vi "Actor Core.vi"(8 "error in":errorcluster, 11 "Sequence Controller in":refnum<class "Sequence Controller.lvclass">) -> (0 "error out":errorcluster, 3 "Actor out":refnum<class "Actor.lvclass">)   [LabVIEW 2024, in "Sequence Controller.lvclass"]
doc: "(<B>Filename</B>: Actor Framework.lvlib:Actor.lvclass:Actor Core.vi)\n\nReceives messages to the actor, reacts to them, and initiates any error handling that may shut the actor down.\n\nDescendant classes may override this VI to append parallel tasks for the actor to complete while it handles messages. Overrides use the Call Parent Method node."
uses:
  Sequence Controller.lvclass
  Sequence Controller.lvclass/Sequence Controller.ctl
  <vilib>/ActorFramework/Actor/Actor.lvclass
  Sequence Elements/Sequence Element Messages/Items Mouse Click Msg/Items Mouse Click Msg.lvclass
  Template Module Messages/Open Item Msg/Open Item Msg.lvclass
  Sequence Controller Messages/Remove Sequence Element Msg/Remove Sequence Element Msg.lvclass
  Process Controller/Process Controller.lvclass
panel:
  in  "Remove Button":bool
  in  "Add Button":bool
  in  "Items":i32(listbox)
  in  "Measure sequence":string(tree)
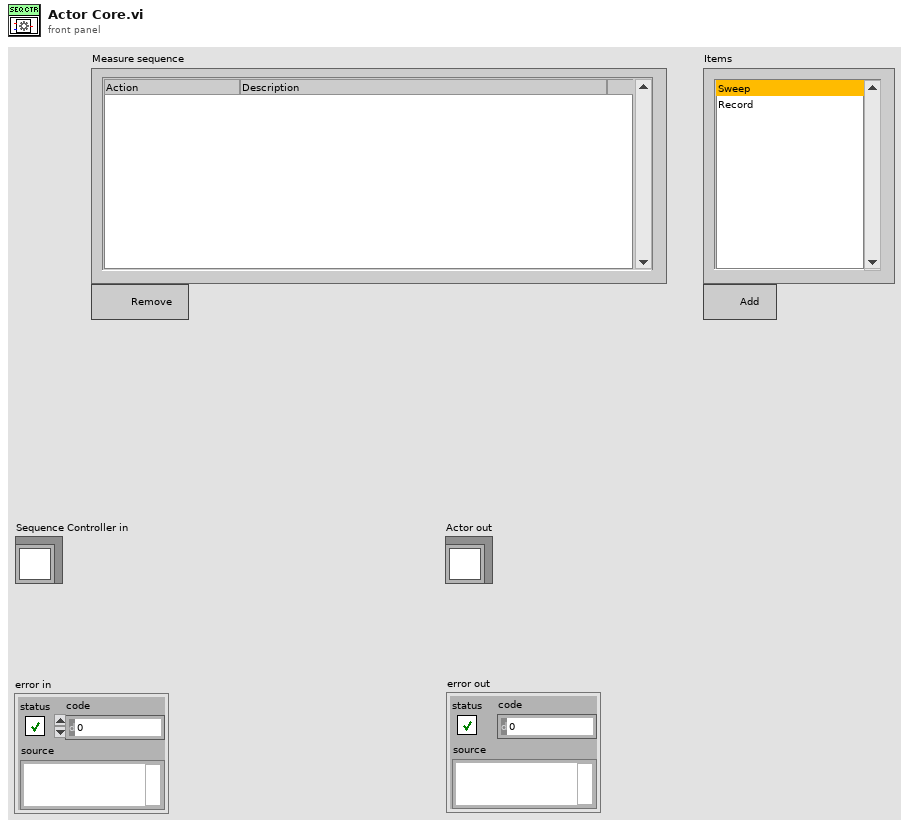
[diagram p1: front panel]
types:
  T1 = typedef "imagedata.ctl" = cluster{"image type":i32, "image depth":i32, "image":u8[], "mask":u8[], "colors":u32[], "Rectangle":cluster{"left":i16, "top":i16, "right":i16, "bottom":i16}}
  T2 = typedef "LVPoint32TypeDef.ctl" = cluster{"Horizontal":i32, "Vertical":i32}
  T3 = cluster{"Shift":bool, "Ctrl":bool, "Alt":bool, "Cmd":bool, "Opt":bool}
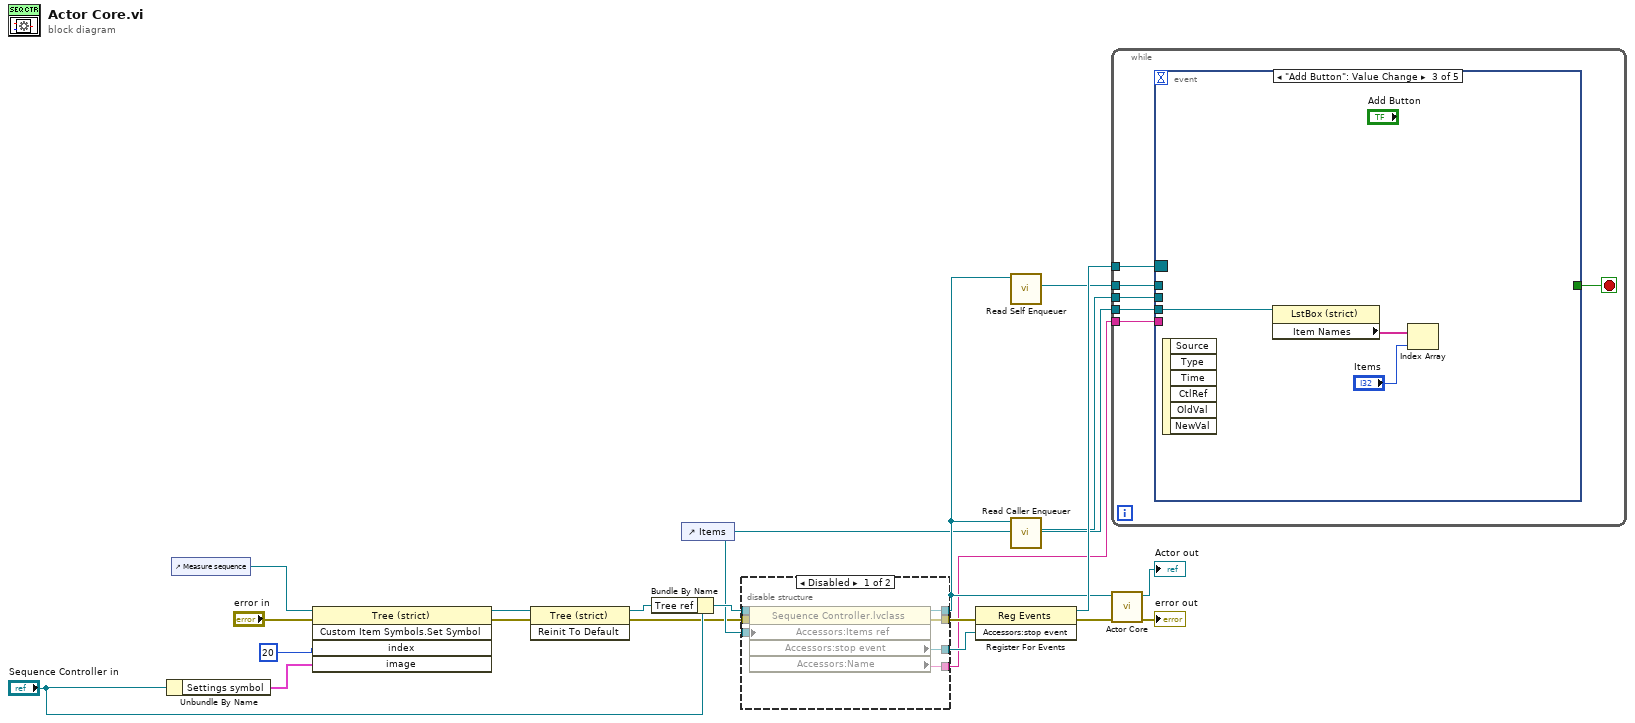
[diagram p0: block diagram]
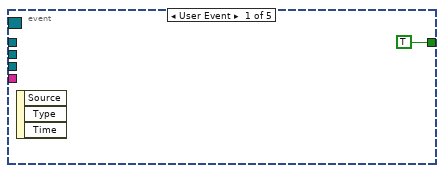
[diagram p3: hidden frame]
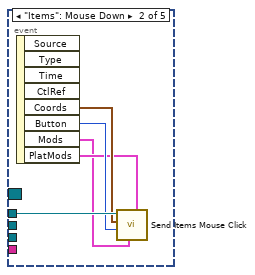
[diagram p4: hidden frame]
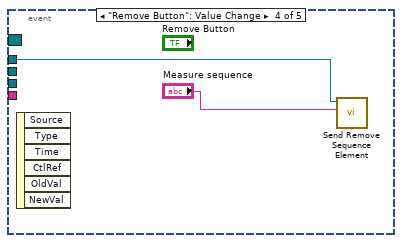
[diagram p5: hidden frame]
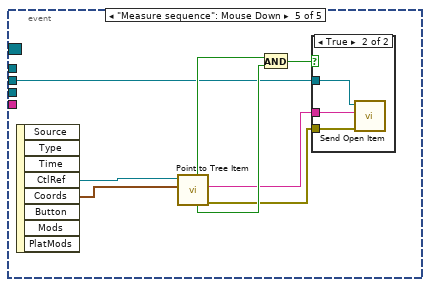
[diagram p6: hidden frame]
diagram:
  n1 = Unbundle By Name("Sequence Controller in") -> ("Settings symbol"=w10:T1)
  n2 = control-ref of="Measure sequence"() -> (w14:refnum<vi>)
  n3 = invoke class="Tree (strict)" method="Custom Item Symbols.Set Symbol"(reference=w14, error in="error in", "index"=20 ("Index"), "image"=w10) -> (reference out=w4:refnum<vi>, error out=w2:errorcluster)  [unwired: 1 in, 3 out]
  n4 = invoke class="Tree (strict)" method="Reinit To Default"(reference=w4, error in=w2) -> (reference out=w3:refnum<vi>, error out=w1:errorcluster)  [unwired: 1 in, 1 out]
  n5 = Bundle By Name(cluster="Sequence Controller in", "Tree ref"=w3) -> (w15:refnum<class "Sequence Controller.lvclass">)
  n6 = control-ref of="Items"() -> (w6:refnum<vi>)
  n7 = disable-structure shown="Disabled" {
    disable-tunnel: [w28 w29] -> w18
    disable-tunnel: w15 -> [w27 w30]
    disable-tunnel: [w26 _] -> w9
    disable-tunnel: [w25 w30] -> w8
    disable-tunnel: w6 -> [w24 _]
    disable-tunnel: [w23 _] -> w5
    disable-tunnel: w1 -> [w22 w29]
    frame Disabled {
      n8 = property class="Sequence Controller.lvclass"(reference=w27, error in=w22, "Accessors:Items ref"=w24) -> (reference out=w25:refnum<class "Sequence Controller.lvclass">, error out=w28:errorcluster, "Accessors:stop event"=w26:refnum<user-event>, "Accessors:Name"=w23:string)
    }
    frame Enabled {
    }
  }
  n9 = register-events(error in=w18, w9) -> (reference out=w19:refnum<event-registration>, error out=w17:errorcluster)  [unwired: 1 in]
  n10 = call <vilib>:"Read Self Enqueuer.vi"("Actor"=w8) -> ("Self Enqueuer"=w16:refnum<class "Message Enqueuer.lvclass">)  [unwired: 10 in]
  n11 = call <vilib>:"Read Caller Enqueuer.vi"("Actor"=w8) -> ("Caller Enqueuer"=w7:refnum<class "Message Enqueuer.lvclass">)  [unwired: 10 in]
  n12 = while {
    tunnel: w19 -> [w36]
    tunnel: w16 -> [w34]
    tunnel: w7 -> [w33]
    tunnel: w6 -> [w32]
    tunnel: w5 -> [w31]
    stop <- w35 stop-if-true
    n13 = event shown="[2] \"Add Button\": Value Change" {
      selector: w36 -> [_ _ _ _ _]
      dyn-events: _ -> [_ _ _ _ _]
      timeout: _ -> [_ _ _ _ _]
      tunnel: [TRUE _ _ _ _] -> w35
      tunnel: w34 -> [_ w42 _ w47 _]
      tunnel: w33 -> [_ _ _ _ w50]
      tunnel: w32 -> [_ _ w45 _ _]
      tunnel: w31 -> [_ _ _ _ _]
      event User Event {
        n14 = event-data() -> ()  [unwired: 1 in, 3 out]
      }
      event "Items": Mouse Down {
        n15 = event-data() -> ("Coords"=w41:T2, "Button"=w40:u16, "Mods"=w38:cluster{"Double Click":bool, "Menu Key":bool}, "PlatMods"=w39:T3)  [unwired: 1 in, 4 out]
        n16 = call "Send Items Mouse Click.vi"("PlatMods"=w39, "Mods"=w38, "Button"=w40, "Coords"=w41, "Message Enqueuer"=w42) -> ()  [unwired: 5 in, 2 out]
      }
      event "Add Button": Value Change {
        n17 = event-data() -> ()  [unwired: 1 in, 6 out]
        n18 = property class="LstBox (strict)"(reference=w45) -> ("Item Names"=w44:string[])  [unwired: 1 in, 2 out]
        n19 = Index Array(array=w44, index="Items") -> ()  [unwired: 1 out]
      }
      event "Remove Button": Value Change {
        n20 = event-data() -> ()  [unwired: 1 in, 6 out]
        n21 = call "Send Remove Sequence Element.vi"("Name"="Measure sequence", "Message Enqueuer"=w47) -> ()  [unwired: 8 in, 2 out]
      }
      event "Measure sequence": Mouse Down {
        n22 = event-data() -> ("CtlRef"=w55:refnum<vi>, "Coords"=w54:T2)  [unwired: 1 in, 6 out]
        n23 = call "Point to Tree Item.vi"("Coords"=w54, "reference"=w55) -> ("Error Out"=w48:errorcluster, "Item"=w49:string, "In Symbol?"=w52:bool, "Valid"=w53:bool)  [unwired: 5 in, 1 out]
        n24 = And(x=w53, y=w52) -> (x .and. y?=w51:bool)
        n25 = case shown="True" w51 {
          tunnel: w50 -> [_ w58]
          tunnel: w49 -> [_ w57]
          tunnel: w48 -> [_ w56]
          frame False {
          }
          frame True {
            n26 = call "Send Open Item.vi"("error in (no error)"=w56, "Item name"=w57, "Message Enqueuer"=w58) -> ()  [unwired: 7 in, 2 out]
          }
        }
      }
    }
  }
  n27 = call-parent "Actor Core.vi"("error in"=w17, "Measure Object in"=w8) -> ("error out"=→"error out":errorcluster, "Actor out"=→"Actor out":refnum<class "Actor.lvclass">)  [unwired: 8 in]
